vi "Configure_Graphs.vi"() -> (4 "Output\nMultiple":dbl[](array[numeric]), 6 "Output\nOffset":dbl[](array[numeric]))   [LabVIEW 2014]
panel:
  in  "Input\nOffset":dbl[](array[numeric])
  in  "Input\nMultiple":dbl[](array[numeric])
  in  "OK Button":bool
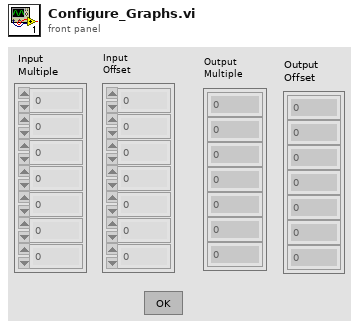
[diagram p1: front panel]
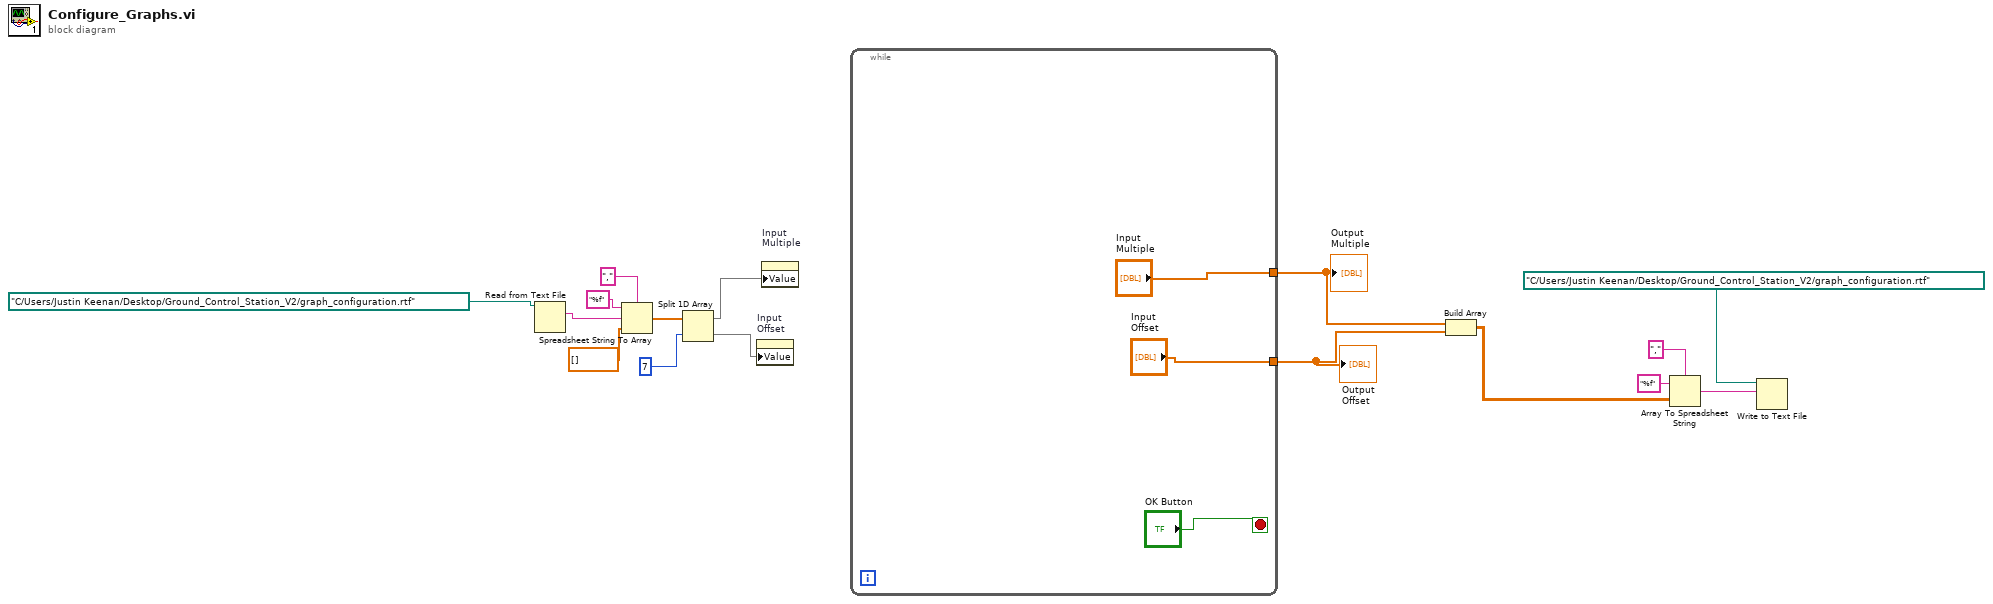
[diagram p0: block diagram]
diagram:
  n1 = Read from Text File(file (use dialog)=path "C:/Users/Justin Keenan/Desktop/Ground_Control_Station_V2/graph_configuration.rtf") -> (text=w11:string)  [unwired: 3 in, 3 out]
  n2 = Spreadsheet String To Array(delimiter (Tab)=",", format string="%f", spreadsheet string=w11, array type (2D Dbl)=dbl[] []) -> (array=w5:dbl[])
  n3 = Split 1D Array(array=w5, index=7) -> (first subarray=w6:dbl[], second subarray=w4:dbl[])
  n4 = property on="Input\nOffset" class="Arr (strict)"("Value"=w4) -> ()  [unwired: 2 in, 2 out]
  n5 = property on="Input\nMultiple" class="Arr (strict)"("Value"=w6) -> ()  [unwired: 2 in, 2 out]
  n6 = while {
    tunnel: ["Input\nMultiple"] -> w3
    tunnel: ["Input\nOffset"] -> w2
    stop <- "OK Button" stop-if-true
  }
  "Output\nMultiple" <- w3
  "Output\nOffset" <- w2
  n7 = Build Array(w3, w2) -> (w1:dbl[][])
  n8 = Array To Spreadsheet String(delimiter (Tab)=",", array=w1, 3:"%f" ("format string")) -> (spreadsheet string=w14:string)
  n9 = Write to Text File(file (use dialog)=path "C:/Users/Justin Keenan/Desktop/Ground_Control_Station_V2/graph_configuration.rtf", text=w14) -> ()  [unwired: 2 in, 3 out]
